vi "Write Channel name.vi"(8 "error in (no error)":errorcluster, 10 "Channel name":string, 11 "Metadata in":refnum<class "Metadata.lvclass">) -> (0 "error out":errorcluster, 3 "Metadata out":refnum<class "Metadata.lvclass">)   [LabVIEW 2020, in "Metadata.lvclass"]
uses:
  Metadata.lvclass
  Metadata.lvclass/Metadata.ctl
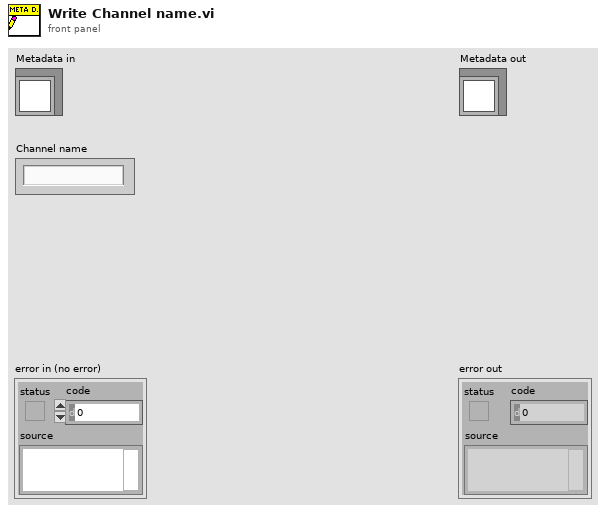
[diagram p1: front panel]
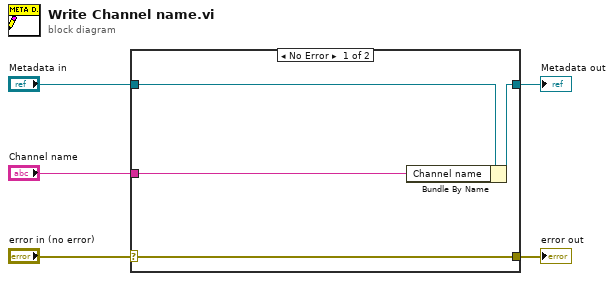
[diagram p0: block diagram]
diagram:
  n1 = case shown="No Error" "error in (no error)" {
    selector: "error in (no error)" -> [w9 w10]
    tunnel: [w9 w10] -> w4
    tunnel: [w7 w11] -> w2
    tunnel: "Metadata in" -> [w8 w11]
    tunnel: "Channel name" -> [w6 _]
    frame No Error {
      n2 = Bundle By Name(cluster=w8, "Channel name"=w6) -> (w7:refnum<class "Metadata.lvclass">)
    }
    frame Error {
    }
  }
  "error out" <- w4
  "Metadata out" <- w2
